vi "Meteo.vi"() -> ()   [LabVIEW 2019]
panel:
  in  "Temp Scale":bool
  in  "Нижний предел":dbl
  in  "Верхний предел":dbl
  out "Температура":dbl(graph)
  in  "?":bool
  out "Предупреждения":string
  # "deg C\n\ndeg F"
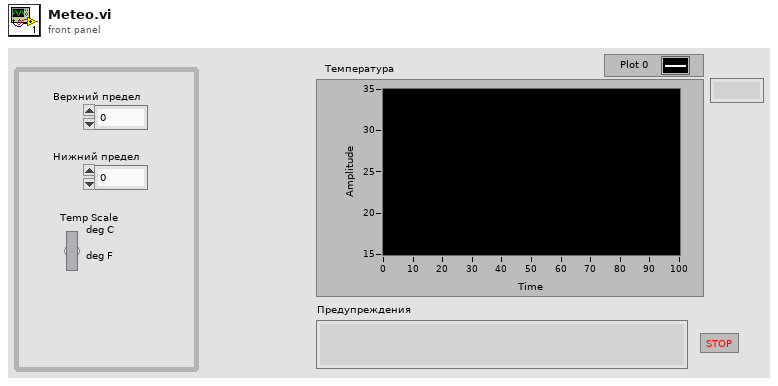
[diagram p1: front panel]
types:
  T1 = enum16{"open", "replace", "create", "open or create", "replace or create", "replace or create with confirmation"}
  T2 = enum16{"Сбор данных", "Анализ", "Сохранение", "Проверка времени"}
  T3 = cluster{"Предупреждение":string, "Нижний предел":dbl, "Верхний предел":dbl, "Температура":dbl}
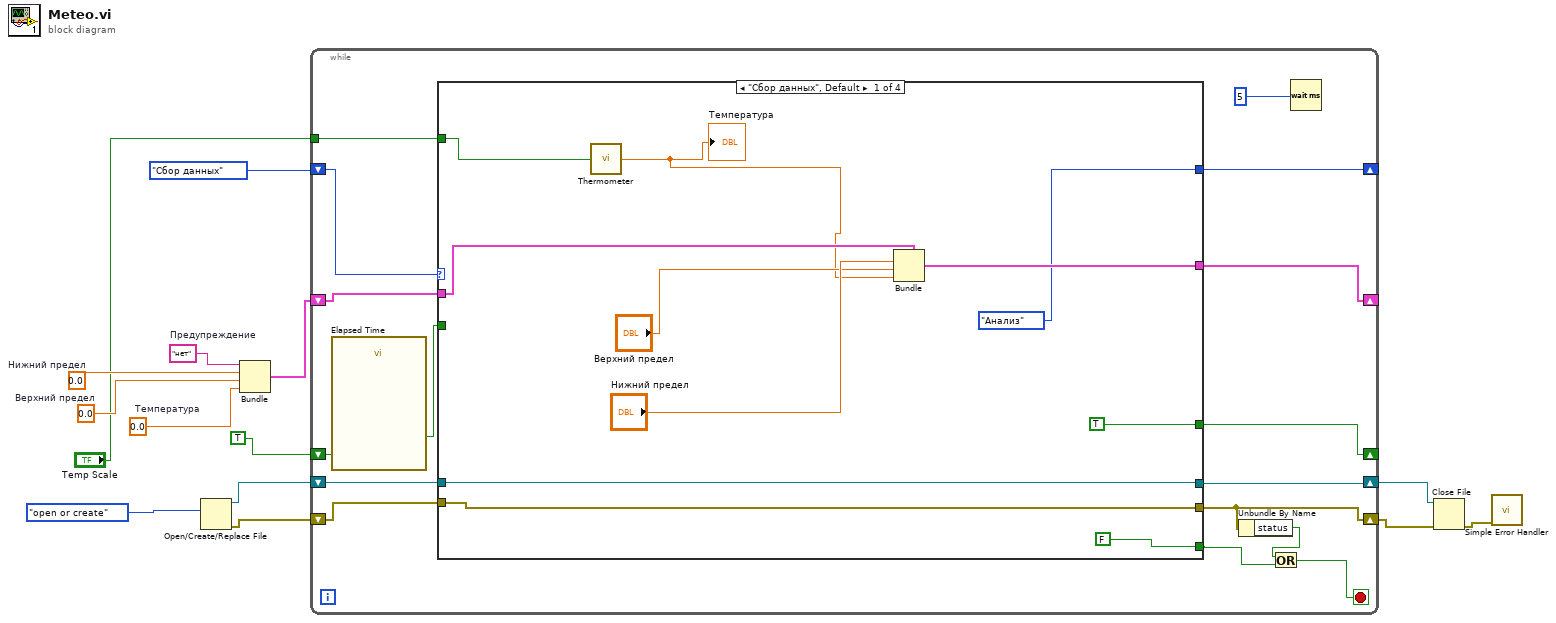
[diagram p0: block diagram]
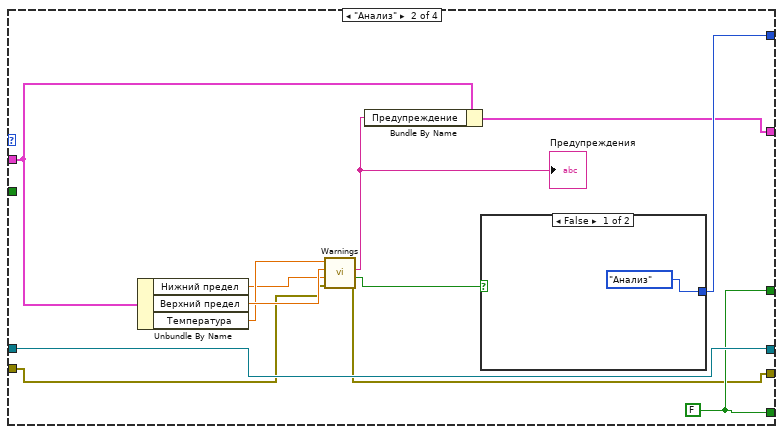
[diagram p2: hidden frame]
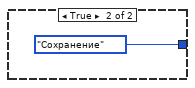
[diagram p3: hidden frame]
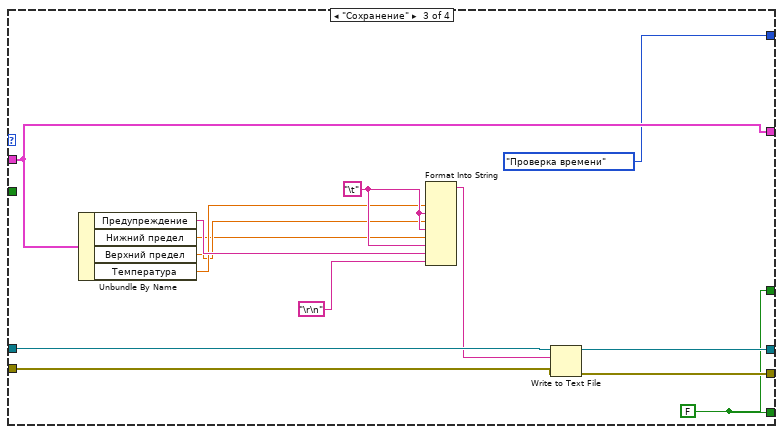
[diagram p4: hidden frame]
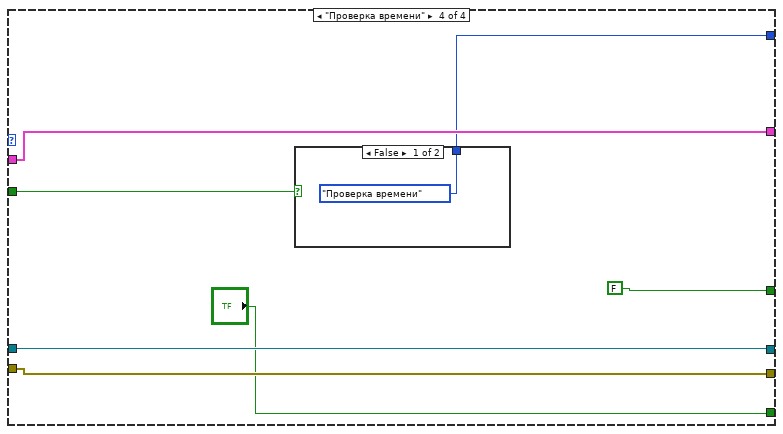
[diagram p5: hidden frame]
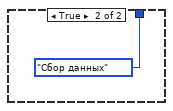
[diagram p6: hidden frame]
diagram:
  w14 = "нет"  # Предупреждение
  w13 = 0.0  # Нижний предел
  w12 = 0.0  # Верхний предел
  w11 = 0.0  # Температура
  n1 = Open/Create/Replace File(operation (0:open)=T1."open or create") -> (refnum out=w7:refnum<file>, error out=w6:errorcluster)  [unwired: 5 in, 1 out]
  n2 = Bundle("Предупреждение"=w14, "Нижний предел"=w13, "Верхний предел"=w12, "Температура"=w11) -> (w10:T3)  [unwired: 1 in]
  n3 = while {
    shift-right: [w22] -> _
    shift-left: w10 -> [w28]
    shift-right: [w27] -> _
    shift-left: T2."Сбор данных" ("Enum") -> [w30]
    shift-right: [w24] -> w4
    shift-left: w7 -> [w26]
    shift-right: [w21] -> w5
    shift-left: w6 -> [w25]
    shift-right: [w16] -> _
    shift-left: TRUE -> [w17]
    tunnel: "Temp Scale" -> [w15]
    stop <- w19 stop-if-true
    n4 = call "Elapsed Time"("Reset"=w17) -> ("Time has Elapsed"=w23:bool)  [unwired: 11 in, 7 out]
    n5 = case shown="\"Сбор данных\", Default" w30 {
      tunnel: w28 -> [w41 w53 w69 w74]
      tunnel: [w40 w46 w69 w74] -> w22
      tunnel: [T2."Анализ" ("Enum") w47 T2."Проверка времени" ("Enum") w72] -> w27
      tunnel: w26 -> [w38 w45 w68 w75]
      tunnel: w25 -> [w37 w43 w67 w76]
      tunnel: [w38 w45 w66 w75] -> w24
      tunnel: [w37 w42 w65 w76] -> w21
      tunnel: w23 -> [_ _ _ w73]
      tunnel: [FALSE w44 w56 "?"] -> w18
      tunnel: [TRUE w44 w56 FALSE] -> w16
      tunnel: w15 -> [w31 _ _ _]
      frame "Сбор данных", Default {
        n6 = call "Thermometer.vi"("Temp Scale"=w31) -> ("Temperature"=w32:dbl)
        "Температура" <- w32
        n7 = Bundle(cluster=w41, "Нижний предел"="Нижний предел", "Верхний предел"="Верхний предел", "Температура"=w32) -> (w40:T3)  [unwired: 1 in]
      }
      frame "Анализ" {
        w44 = FALSE
        n8 = Unbundle By Name(w53) -> ("Нижний предел"=w50:dbl, "Верхний предел"=w52:dbl, "Температура"=w51:dbl)
        n9 = call "Warnings.vi"("error in (no error)"=w43, "Минимальная"=w50, "Максимальная"=w52, "Текущая"=w51) -> ("error out"=w42:errorcluster, "Предупреждение"=w48:bool, "Текст"=w49:string)  [unwired: 5 in]
        "Предупреждения" <- w49
        n10 = Bundle By Name(cluster=w53, "Предупреждение"=w49) -> (w46:T3)
        n11 = case shown="False" w48 {
          tunnel: [T2."Анализ" ("Enum") T2."Сохранение" ("Enum")] -> w47
          frame False {
          }
          frame True {
          }
        }
      }
      frame "Сохранение" {
        w56 = FALSE
        w60 = "\t"
        n12 = Unbundle By Name(w69) -> ("Предупреждение"=w62:string, "Нижний предел"=w57:dbl, "Верхний предел"=w58:dbl, "Температура"=w59:dbl)
        n13 = Format Into String(w59, w60, w58, w60, w57, w60, w62, "\r\n") -> (resulting string=w63:string)  [unwired: 3 in, 1 out]
        n14 = Write to Text File(file (use dialog)=w68, text=w63, error in=w67) -> (refnum out=w66:refnum<file>, error out=w65:errorcluster)  [unwired: 1 in, 1 out]
      }
      frame "Проверка времени" {
        n15 = case shown="False" w73 {
          tunnel: [T2."Проверка времени" ("Enum") T2."Сбор данных" ("Enum")] -> w72
          frame False {
          }
          frame True {
          }
        }
      }
    }
    n16 = Unbundle By Name(w21) -> ("status"=w20:bool)
    n17 = Or(x=w20, y=w18) -> (x .or. y?=w19:bool)
    n18 = Wait (ms)(milliseconds to wait=5) -> ()  [unwired: 1 out]
  }
  n19 = Close File(refnum=w4, error in=w5) -> (error out=w3:errorcluster)  [unwired: 1 out]
  n20 = call <vilib>:"Simple Error Handler.vi"("error in (no error)"=w3) -> ()  [unwired: 4 in, 5 out]
